vi "ClientGUISingleLine.vi"() -> ()   [LabVIEW 2021]
doc: "Le protocole UDP diffère du protocole TCP car il n'y a pas de détection d'erreur avec les paquets d'informations qui sont envoyés ; il n'y a donc aucune garantie qu'un destinataire reçoive bien des données.\n\nLe protocole UDP offre la possibilité de diffuser des données sur un réseau. Spécifiez simplement une adresse IP de uns (255.255.255.255) pour essayer de diffuser l'information sur tout le réseau. Gardez à l'esprit que des routeurs et d'autres périphériques de réseau refusent généralement de diffuser au-delà de certains points, la diffusion est donc limitée dans la pratique."
panel:
  out "?":u8(graph)
  in  "Value In":u8=1 caption="PWM Write [0 - 255]"
  out "Current PWM":u8
  in  "Période\n(en ds)":u32(slide)=100 min=5 max=100 step=5 scale=5.0..100.0
  in  "?":bool
  in  "Pin":u8=1 caption="Pin [0 - 11]" max=11
  out "Analog Read":u16
  out "?":u16(graph)
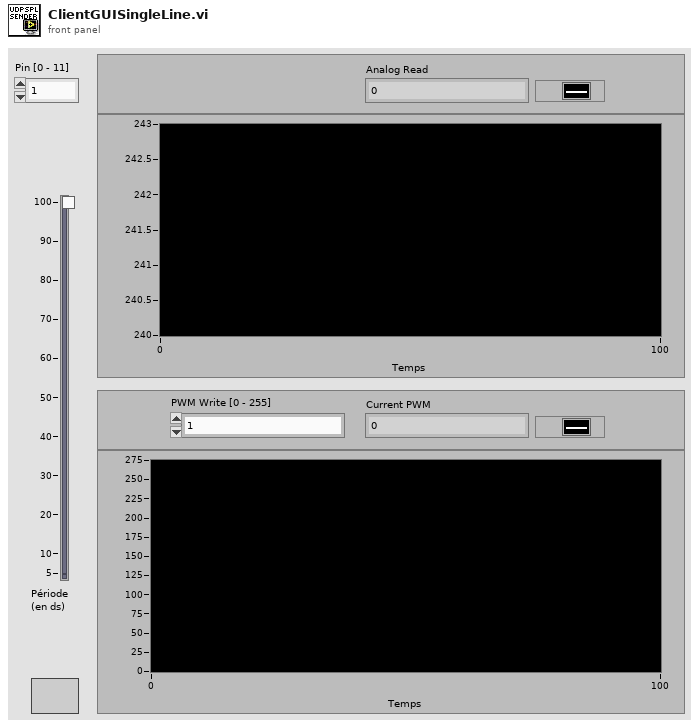
[diagram p1: front panel]
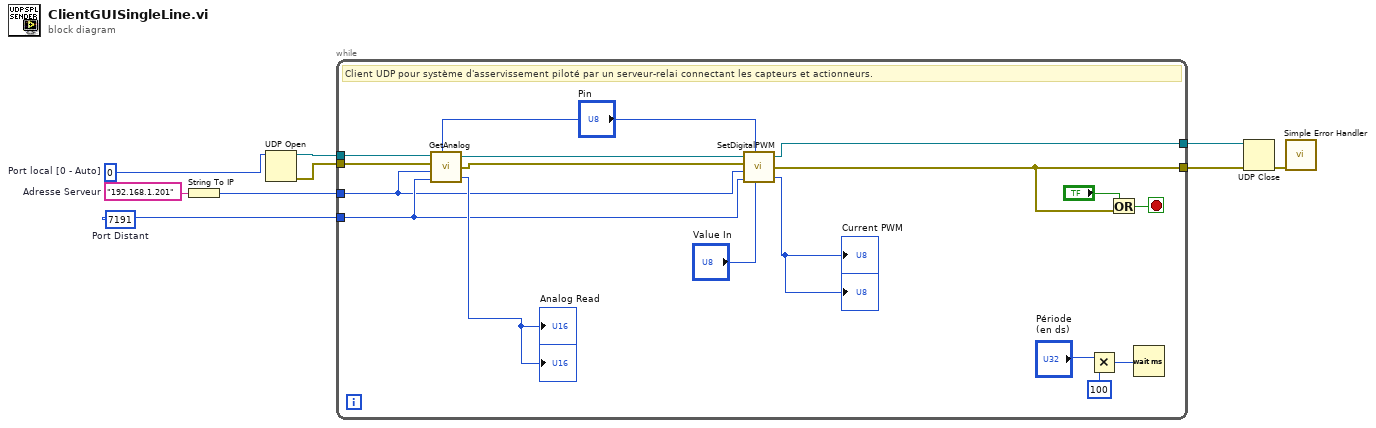
[diagram p0: block diagram]
diagram:
  w2 = u16 7191  # Port Distant
  w6 = u16 0  # Port local [0 - Auto]
  w9 = "192.168.1.201"  # Adresse Serveur
  n1 = String To IP(1:w9) -> (0:w1:u32)
  n2 = UDP Open(11:w6) -> (port=w8:refnum<k16>, 0:w7:errorcluster)  [unwired: 4 in, 1 out]
  n3 = while {
    tunnel: w8 -> [w22]
    tunnel: w7 -> [w21]
    tunnel: [w14] -> w5
    tunnel: w1 -> [w15]
    tunnel: w2 -> [w16]
    tunnel: [w13] -> w3
    stop <- w19 stop-if-true
    # "Client UDP pour système d'asservissement piloté par un serveur-relai connectant les capteurs et actionneurs."
    n4 = call "GetAnalog.vi"("Connexion réseau UDP en entrée"=w22, "Pin"="Pin", "entrée d'erreur (pas d'erreur)"=w21, "Adresse IP"=w15, "Port Distant"=w16) -> ("Connexion réseau UDP en sortie"=w18:refnum<k16>, "sortie d'erreur"=w17:errorcluster, "Return Value"=→"?" →"Analog Read":u16)  [unwired: 1 in]
    n5 = call "SetDigitalPWM.vi"("Connexion réseau UDP en entrée"=w18, "Pin"="Pin", "entrée d'erreur (pas d'erreur)"=w17, "Adresse IP"=w15, "Value In"="Value In", "Port Distant"=w16) -> ("Connexion réseau UDP en sortie"=w14:refnum<k16>, "error out"=w13:errorcluster, "Return Value"=→"?" →"Current PWM":u8)
    n6 = Multiply(x="Période\n(en ds)", y=u32 100) -> (x*y=w25:u32)
    n7 = Or(x="?", y=w13) -> (x .or. y?=w19:bool)
    n8 = Wait (ms)(milliseconds to wait=w25) -> ()  [unwired: 1 out]
  }
  n9 = UDP Close(connection ID=w5, 8:w3) -> (error out=w4:errorcluster)  [unwired: 1 out]
  n10 = call <vilib>:"Simple Error Handler.vi"("error in (no error)"=w4) -> ()  [unwired: 4 in, 5 out]
